vi "Deluxeglobal.vi"() -> ()   [LabVIEW 2024]
panel:
  in  "Deluxe":bool
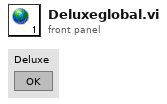
[diagram p1: front panel]
diagram:
